vi "Read XML Results.vi"(8 "error in":errorcluster, 11 "XML Path":path) -> (0 "error out":errorcluster, 3 "Changes":i32[](array[numeric]) caption="0-Front Panel\n1-Block Diagram\n2-Attribute")   [LabVIEW 2020, in "Peer Review.lvclass"]
uses:
  Peer Review.lvclass
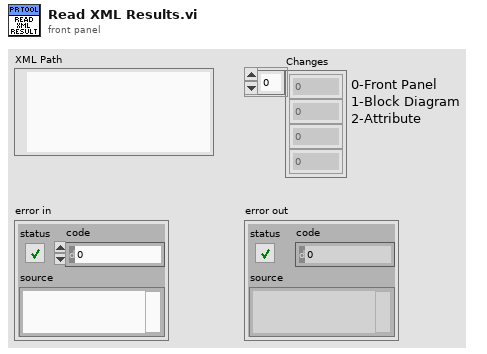
[diagram p1: front panel]
types:
  T1 = enum16{"open", "replace", "create", "open or create", "replace or create", "replace or create with confirmation"}
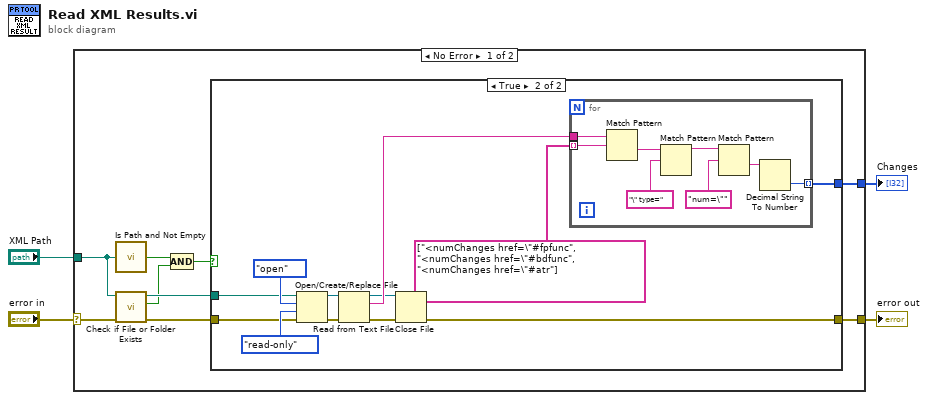
[diagram p0: block diagram]
diagram:
  n1 = case shown="No Error" "error in" {
    selector: "error in" -> [w11 w35]
    tunnel: [w13 _] -> w4
    tunnel: [w12 w35] -> w3
    tunnel: "XML Path" -> [w8 _]
    frame No Error {
      n2 = call <vilib>:"Is Path and Not Empty.vi"("path"=w8) -> ("Is Path and Not Empty?"=w7:bool)  [unwired: 4 in]
      n3 = call <vilib>:"Check if File or Folder Exists.vi"("error in (no error)"=w11, "path"=w8) -> ("error out"=w10:errorcluster, "file or folder exists?"=w6:bool, "dup path"=w9:path)  [unwired: 7 in]
      n4 = Compound Arithmetic op=AND(w7, w6) -> (w5:bool)
      n5 = case shown="True" w5 {
        tunnel: [_ w25] -> w13
        tunnel: [w14 w17] -> w12
        tunnel: w9 -> [_ w15]
        tunnel: w10 -> [w14 w16]
        frame False {
        }
        frame True {
          n6 = Open/Create/Replace File(file path (use dialog)=w15, error in=w16, operation (0:open)=T1."open", access (0:read/write)=enum16{"read/write", "read-only", "write-only"}."read-only") -> (refnum out=w21:refnum<file>, error out=w22:errorcluster)  [unwired: 2 in, 1 out]
          n7 = Read from Text File(file (use dialog)=w21, error in=w22) -> (refnum out=w19:refnum<file>, text=w20:string, error out=w18:errorcluster)  [unwired: 2 in, 1 out]
          n8 = Close File(refnum=w19, error in=w18) -> (error out=w17:errorcluster)  [unwired: 1 out]
          n9 = for {
            tunnel: w20 -> [w34]
            tunnel: string[] ["<numChanges href=\"#fpfunc", "<numChanges href=\"#bdfunc", "<numChanges href=\"#atr"] ("regular expression") -> [w33] mode=indexing
            tunnel: [w27] -> w25 mode=indexing
            n10 = Match Pattern(string=w34, regular expression=w33) -> (after substring=w32:string)  [unwired: 1 in, 3 out]
            n11 = Match Pattern(string=w32, regular expression="\" type=") -> (before substring=w29:string)  [unwired: 1 in, 3 out]
            n12 = Match Pattern(string=w29, regular expression="num=\"") -> (after substring=w28:string)  [unwired: 1 in, 3 out]
            n13 = Decimal String To Number(string=w28) -> (number=w27:i32)  [unwired: 2 in, 1 out]
          }
        }
      }
    }
    frame Error {
    }
  }
  "error out" <- w3
  "Changes" <- w4
